vi "compare-trapezoid-profile-PID-position-ctrl.vi"() -> ()   [LabVIEW 2019]
uses:
  Secret_Control_Library_Protected/CtrlTrain_Pos_ctrl_TuningParameters.ctl
  <vilib>/Rock Robotics/WPI/ThirdParty/JAS_Junk/TrajLib/SlewRateLimiter_New.vi
  <vilib>/Rock Robotics/WPI/ThirdParty/JAS_Junk/TrajLib/SlewRateLimiter_Reset.vi
  <vilib>/Rock Robotics/WPI/ThirdParty/JAS_Junk/TrajLib/SlewRateLimiter_Calculate.vi
  <vilib>/Rock Robotics/WPI/ThirdParty/JAS_Junk/TrajLib/SlewRateLimiter_SetRate.vi
  <vilib>/Rock Robotics/WPI/ThirdParty/JAS_Junk/TrajLib/ProfiledPIDController_SetPID.vi
  <vilib>/Rock Robotics/WPI/ThirdParty/JAS_Junk/TrajLib/ProfiledPIDController_SetIntegratorRange.vi
  <vilib>/Rock Robotics/WPI/ThirdParty/JAS_Junk/TrajLib/ProfiledPIDController_SetTolerance_PosVel.vi
  <vilib>/Rock Robotics/WPI/ThirdParty/JAS_Junk/TrajLib/ProfiledPIDController_DisableContInput.vi
  <vilib>/Rock Robotics/WPI/ThirdParty/JAS_Junk/TrajLib/ProfiledPIDController_EnableContInput.vi
  <vilib>/Rock Robotics/WPI/ThirdParty/JAS_Junk/TrajLib/ProfiledPIDController_Reset_PosOnly.vi
  <vilib>/Rock Robotics/WPI/ThirdParty/JAS_Junk/TrajLib/ProfiledPIDController_NewPeriod.vi
  <vilib>/Rock Robotics/WPI/ThirdParty/JAS_Junk/TrajLib/ProfiledPIDController_Calculate_Meas_Goal.vi
  <vilib>/Rock Robotics/WPI/ThirdParty/JAS_Junk/TrajLib/ProfiledPIDController_AtGoal.vi
  <vilib>/Rock Robotics/WPI/ThirdParty/JAS_Junk/TrajLib/ProfiledPIDController_AtSetpoint.vi
  <vilib>/Rock Robotics/WPI/ThirdParty/JAS_Junk/TrajLib/ProfiledPIDController_SetConstraints.vi
  <vilib>/Rock Robotics/WPI/ThirdParty/JAS_Junk/TrajLib/Util_GetTime.vi
  <vilib>/Rock Robotics/WPI/ThirdParty/JAS_Junk/TrajLib/PIDController_SetPID.vi
  <vilib>/Rock Robotics/WPI/ThirdParty/JAS_Junk/TrajLib/PIDController_SetIntegratorRange.vi
  <vilib>/Rock Robotics/WPI/ThirdParty/JAS_Junk/TrajLib/PIDController_SetTolerancePandV.vi
  <vilib>/Rock Robotics/WPI/ThirdParty/JAS_Junk/TrajLib/PIDController_DisableContinousInput.vi
  <vilib>/Rock Robotics/WPI/ThirdParty/JAS_Junk/TrajLib/PIDController_EnableContinousInput.vi
  <vilib>/Rock Robotics/WPI/ThirdParty/JAS_Junk/TrajLib/TrapProfState_New.vi
  <vilib>/Rock Robotics/WPI/ThirdParty/JAS_Junk/TrajLib/ProfiledPIDController_Reset.vi
  <vilib>/Rock Robotics/WPI/ThirdParty/JAS_Junk/TrajLib/PIDController_NewPeriod.vi
  <vilib>/Rock Robotics/SystemInterfaces/NetworkCommunication/NetComm_UsageReport_report.vi
  <vilib>/Rock Robotics/WPI/ThirdParty/JAS_Junk/TrajLib/ProfiledPIDController_SetGoal_PosOnly.vi
  <vilib>/Rock Robotics/WPI/ThirdParty/JAS_Junk/TrajLib/ProfiledPIDController_Calculate_Meas.vi
  <vilib>/Rock Robotics/WPI/ThirdParty/JAS_Junk/TrajLib/TrapProfState_Equals.vi
  <vilib>/Rock Robotics/WPI/ThirdParty/JAS_Junk/TrajLib/PIDController_AtSetpoint.vi
  <vilib>/Rock Robotics/WPI/ThirdParty/JAS_Junk/TrajLib/VI/Util_GetTime_U32.vi
  <vilib>/Rock Robotics/WPI/ThirdParty/JAS_Junk/TrajLib/PIDController_Reset.vi
  <vilib>/Rock Robotics/WPI/ThirdParty/JAS_Junk/TrajLib/ProfiledPIDController_SetGoal.vi
  <vilib>/Rock Robotics/WPI/ThirdParty/JAS_Junk/TrajLib/PIDController_Calculate_SP_PV.vi
  <vilib>/Rock Robotics/WPI/ThirdParty/JAS_Junk/TrajLib/TrapProfile_New.vi
  <vilib>/Rock Robotics/WPI/ThirdParty/JAS_Junk/TrajLib/ProfiledPIDController_GetPeriod.vi
  <vilib>/Rock Robotics/WPI/ThirdParty/JAS_Junk/TrajLib/TrapProfile_Calculate.vi
  <vilib>/Rock Robotics/WPI/ThirdParty/JAS_Junk/TrajLib/ControllerUtil_GetModulusError.vi
  <vilib>/Rock Robotics/WPI/ThirdParty/JAS_Junk/TrajLib/PIDController_SetSetpoint.vi
  <vilib>/Rock Robotics/WPI/ThirdParty/JAS_Junk/TrajLib/PIDController_Calculate_PV.vi
  <vilib>/Rock Robotics/WPI/ThirdParty/JAS_Junk/TrajLib/TrapProfile_ShouldFlipAcceleration.vi
  <vilib>/Rock Robotics/WPI/ThirdParty/JAS_Junk/TrajLib/TrapProfile_Direct.vi
  <vilib>/Rock Robotics/WPI/ThirdParty/JAS_Junk/TrajLib/PIDController_GetPeriod.vi
  <vilib>/addons/control/pid/pid.llb/PID Lead-Lag (DBL).vi
  <vilib>/Rock Robotics/WPI/ThirdParty/JAS_Junk/TrajLib/Globals/Util_LibraryGlobals.vi
  <vilib>/Rock Robotics/WPI/ThirdParty/JAS_Junk/TrajLib/VI/Util_GetTime_U64.vi
  <vilib>/addons/control/pid/NI_PID_pid.lvlib
  Secret_Control_Library_Protected/Secret_Control_Library_Protected.lvlib
  <vilib>/Rock Robotics/WPI/ThirdParty/JAS_Junk/TrajLib/Trajectory_Library.lvlib
panel:
  in  "Tab Control":T1(tab)
  out "PC-SP, PV, CO Chart":T2(graph)
  in  "Desired Position":dbl(slide) min=0.0 max=90.0 scale=0.0..90.0
  in  "Auto - Set Position To 0 / Manual - Lower":bool
  in  "Auto - Set Position to 90 / Manual - Raise":bool
  in  "Set Position to Desired\n(Select to activate position)":bool
  out "Selected Setpoint \n(In Manual \ntracks Position)":dbl
  out "Trap-Current \nPosition 2":dbl format="%.2f"
  out "Trap-Motor \nDemand2":dbl format="%#.2f"
  out "Trap-Position Error":dbl format="%#3.2f"
  out "Trap-SP, PV, CO Chart":T2(graph)
  out "Trap-Current Position":dbl(knob) scale=-10.0..100.0
  in  "Auto / Manual":bool=TRUE
  in  "MinLimitSwitch":bool
  in  "MaxLimitSwitch":bool
  out "Trap-In Position":bool
  out "PC-Current \nPosition 2":dbl format="%.2f"
  out "PC-Motor \nDemand 2":dbl format="%#.2f"
  out "PC-Current Position 3":dbl(knob) scale=-10.0..100.0
  out "Selected Setpoint \n(In Manual \ntracks Position) 2":dbl
  out "PC-In Position":bool
  out "PC-Position Error":dbl format="%#3.2f"
  in  "MaxLimitSwitch 2":bool
  in  "MinLimitSwitch 2":bool
  out "AtGoal":bool
  in  "Trap-Max Accel":dbl=18.0 format="%#_13g"
  in  "PC-TuningParameters":T3={"MaxOutput"=1.0, "MinOutput"=0.25, "PositionErrThreshold"=6.0, "PositionErrDeadband"=0.5, "ReverseOutput"=FALSE, "PositionMax"=89.0, "PositionMin"=1.0, "WithinDBCount"=5} {"WithinDBCount" min=1}
  in  "trap-PositionTolerance":dbl=0.5 format="%#_13g"
  in  "Trap-VelocityTolerance":dbl=1.0 format="%#_13g"
  in  "Trap-ConsecutiveAtGoalCount":i32=5
  in  "Trap-Max Speed":dbl=8.5 format="%#_13g"
  in  "PC-MaxAccelRate":dbl=1.4 format="%#_13g"
  in  "Output Deadband":dbl=0.08 format="%#_13g"
  in  "At Reference Count":i32=10
  in  "Max Allowd Position":dbl=89.0 format="%#_13g"
  in  "Min Allowd Position":dbl=1.0 format="%#_13g"
  in  "ErrorThreshold":dbl=6.5 format="%#_13g"
  in  "MaxOutput":dbl=1.0 format="%#_13g"
  in  "Output Threshold":dbl=1.0 format="%#_13g"
  in  "ErrorDeadband":dbl=0.5 format="%#_13g"
  in  "Kp":dbl=1.5 format="%#_13g"
  out "Both-Current-Setpoint":dbl
  out "Trap-Current-Position":dbl
  out "Both-Manual-Lower":bool
  out "Both-Manual-Raise":bool
  out "Trap-Motor-Demand":dbl
  out "PC-Current-Position":dbl
  out "PC-Motor-Demand":dbl
  # "Compare trapezoid with position control"
  # "Toggle these switches to simulate a limit switch input."
  # "Trapezoid Profile"
  # "Position Control"
  # "Max Vel = 8.5"
  # "Max Output = 1.0"
  # "1.25"
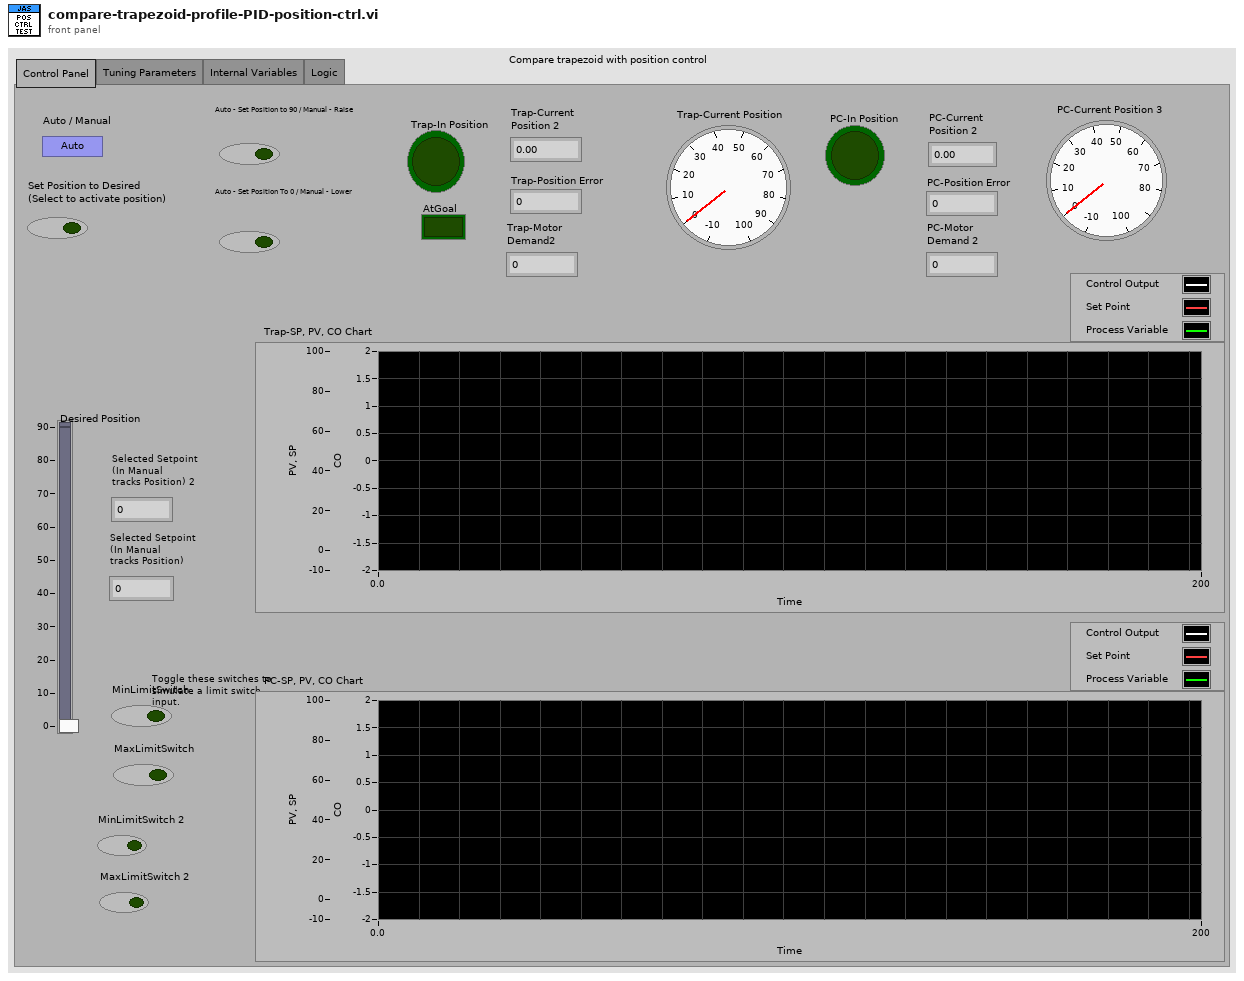
[diagram p1: front panel]
types:
  T1 = enum32{"Control Panel", "Tuning Parameters", "Internal Variables", "Logic"}
  T2 = cluster{"MotorDemand":dbl, "CurrentSetpoint":dbl, "CurrentPosition":dbl}
  T3 = typedef "Secret_Control_Library_Protected.lvlib/CtrlTrain_Pos_ctrl_TuningParameters.ctl" = cluster{"MaxOutput":dbl, "MinOutput":dbl, "PositionErrThreshold":dbl, "PositionErrDeadband":dbl, "ReverseOutput":bool, "PositionMax":dbl, "PositionMin":dbl, "WithinDBCount":i32}
  T4 = cluster{"gain":dbl, "lag time":dbl, "lead time":dbl}
  T5 = cluster{"PC-Motor-Demand":dbl, "Both-Current-Setpoint":dbl, "PC-Current-Position":dbl}
  T6 = typedef "Trajectory_Library.lvlib/PID_TUNING.ctl" = cluster{"Kp":dbl, "Ki":dbl, "Kd":dbl, "MaximumIntegral":dbl, "MinimumIntegral":dbl}
  T7 = typedef "Trajectory_Library.lvlib/PID_INPUT_LIMITS.ctl" = cluster{"MaxInput":dbl, "MinInput":dbl, "Continuous":bool}
  T8 = typedef "Trajectory_Library.lvlib/TRAPEZOID_PROFILE_CONSTRAINT.ctl" = cluster{"MaxVelocity":dbl, "MaxAcceleration":dbl}
  T9 = typedef "Trajectory_Library.lvlib/PID_ERROR_TOLERANCE.ctl" = cluster{"PositionTolerance":dbl, "VelocityTolerance":dbl}
  T10 = typedef "Trajectory_Library.lvlib/PROFILED_PID_CONTROLLER.ctl" = cluster{"Controller":T11, "Goal":T12, "Setpoint":T12, "Constraint":T8}
  T11 = typedef "Trajectory_Library.lvlib/PID_CONTROLLER.ctl" = cluster{"Kp":dbl, "Ki":dbl, "Kd":dbl, "Period":dbl, "Max_Integral":dbl, "Min_Integral":dbl, "Max_Input":dbl, "Min_Input":dbl, "Continuous":bool, "PositionError":dbl, "VelocityError":dbl, "PrevError":dbl, "TotalError":dbl, "PositionTolerance":dbl, "VelocityTolerance":dbl, "SetPoint":dbl, "Kf":dbl, "Prev_Deriv":dbl, "Prev_Deriv 2":dbl, "DerivativeFilter":bool, "Min_Output":dbl, "Max_Output":dbl, "Prev_F_P":dbl, "Prev_F_P_2":dbl, "AntiWindupActive":bool, "Measurement":dbl}
  T12 = typedef "Trajectory_Library.lvlib/TRAPEZOID_PROFILE_STATE.ctl" = cluster{"Position":dbl, "Velocity":dbl}
  T13 = cluster{"Trap-Motor-Demand":dbl, "Both-Current-Setpoint":dbl, "Trap-Current-Position":dbl}
  T14 = typedef "Trajectory_Library.lvlib/PosCtrl_Tuning_Type.ctl" = cluster{"Slope":dbl, "Offset":dbl, "Error Deadband":dbl, "At Reference Count":i32, "Negate Output":bool, "Max Allowd Position":dbl, "Min Allowd Position":dbl}
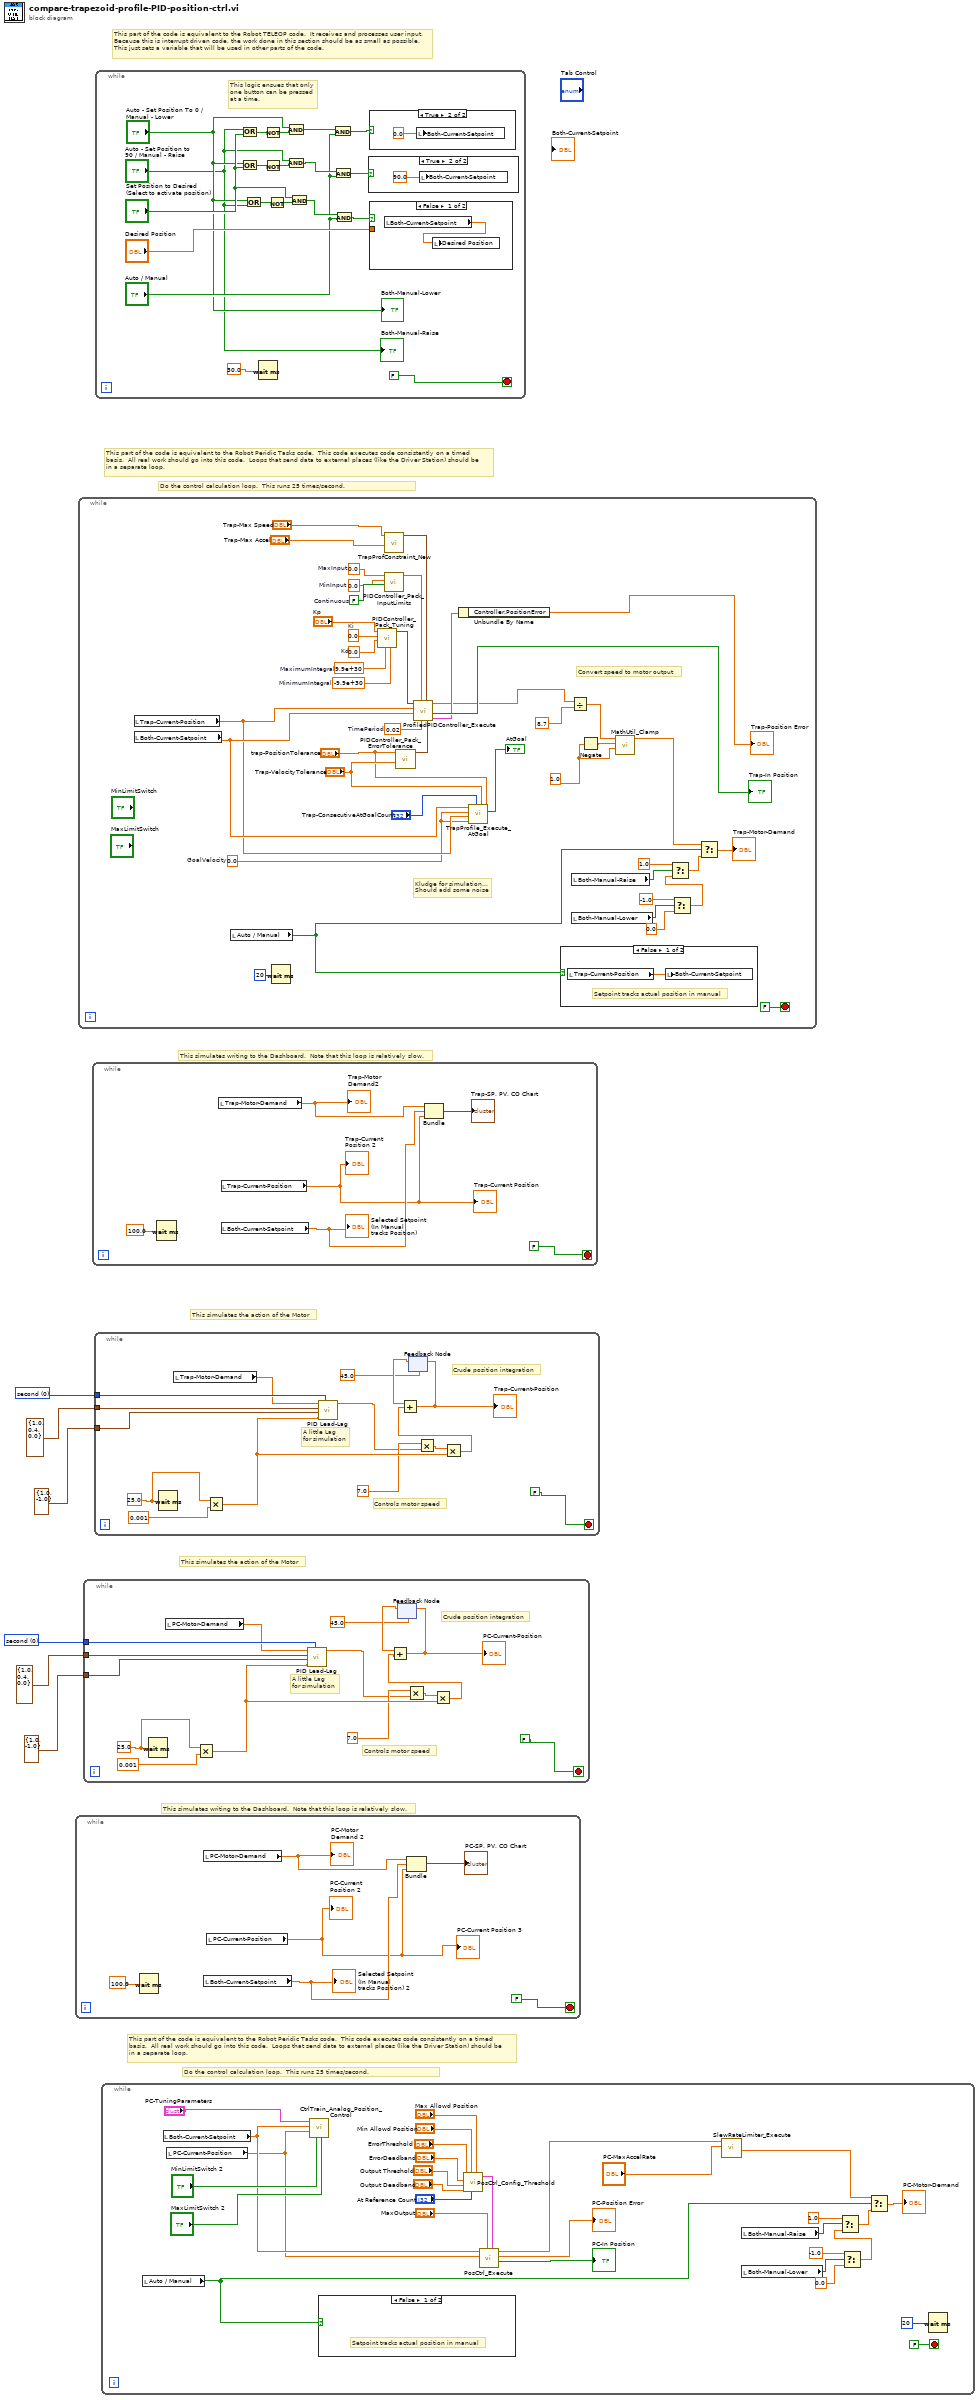
[diagram p0: block diagram]
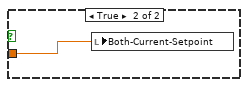
[diagram p4: hidden frame]
diagram:
  w1 = u16 0 items=["second", "minute"] ("time unit")
  w6 = u16 0 items=["second", "minute"] ("time unit")
  # "Do the control calculation loop.  This runs 25 times/second."
  # "This part of the code is equivalent to the Robot Peridic Tasks code.  This code executes code consistently on a timed\nbasis.  All real work should go into this code.  Loops that send data to external places (like the Driver Station) should be \nin a separate loop."
  # "This simulates writing to the Dashboard.  Note that this loop is relatively slow."
  # "This simulates the action of the Motor"
  # "This simulates the action of the Motor"
  # "This simulates writing to the Dashboard.  Note that this loop is relatively slow."
  # "Do the control calculation loop.  This runs 25 times/second."
  # "This part of the code is equivalent to the Robot Peridic Tasks code.  This code executes code consistently on a timed\nbasis.  All real work should go into this code.  Loops that send data to external places (like the Driver Station) should be \nin a separate loop."
  # "This part of the code is equivalent to the Robot TELEOP code.  It receives and processes user input.\nBecause this is interrupt driven code, the work done in this section should be as small as possible.\nThis just sets a variable that will be used in other parts of the code."
  n1 = while {
    stop <- FALSE stop-if-true
    n2 = Wait (ms)(milliseconds to wait=100.0) -> ()  [unwired: 1 out]
    n3 = local read "PC-Motor-Demand"() -> (w8:dbl)
    "PC-Motor \nDemand 2" <- w8
    n4 = local read "Both-Current-Setpoint"() -> (w10:dbl)
    "Selected Setpoint \n(In Manual \ntracks Position) 2" <- w10
    n5 = local read "PC-Current-Position"() -> (w9:dbl)
    "PC-Current \nPosition 2" <- w9
    "PC-Current Position 3" <- w9
    n6 = Bundle("PC-Motor-Demand"=w8, "Both-Current-Setpoint"=w10, "PC-Current-Position"=w9) -> (→"PC-SP, PV, CO Chart":T5)  [unwired: 1 in]
  }
  n7 = while {
    stop <- FALSE stop-if-true
    w23 = 1.0
    w37 = 0.0  # MaxInput
    w38 = 0.0  # MinInput
    w39 = FALSE  # Continuous
    w33 = 0.0  # Ki
    w34 = 0.0  # Kd
    w35 = 9.9e+30  # MaximumIntegral
    w36 = -9.9e+30  # MinimumIntegral
    w13 = 0.0  # GoalVelocity
    w31 = 0.02  # TimePeriod
    # "Convert speed to motor output"
    # "Kludge for simulation...\nShould add some noise"
    n8 = local read "Trap-Current-Position"() -> (w15:dbl)
    n9 = local read "Both-Current-Setpoint"() -> (w16:dbl)
    n10 = local read "Auto / Manual"() -> (w49:bool)
    n11 = Wait (ms)(milliseconds to wait=u32 20) -> ()  [unwired: 1 out]
    n12 = call <vilib>:"PIDController_Pack_Tuning.vi"("MinimumIntegral"=w36, "MaximumIntegral"=w35, "Kd"=w34, "Ki"=w33, "Kp"="Kp") -> ("PID Tuning"=w41:T6)  [unwired: 6 in]
    n13 = call <vilib>:"PIDController_Pack_InputLimits.vi"("Continuous"=w39, "MinInput"=w38, "MaxInput"=w37) -> ("PID Input Limits"=w42:T7)  [unwired: 8 in]
    n14 = call <vilib>:"TrapProfConstraint_New.vi"("Max Accel"="Trap-Max Accel", "Max Speed (M/S)"="Trap-Max Speed") -> ("TRAPEZOID_PROFILE_CONSTRAINT"=w40:T8)  [unwired: 9 in]
    n15 = call <vilib>:"PIDController_Pack_ErrorTolerance.vi"("VelocityTolerance"="Trap-VelocityTolerance", "PositionTolerance"="trap-PositionTolerance") -> ("PID Error Tolerance"=w30:T9)  [unwired: 9 in]
    n16 = call <vilib>:"ProfiledPIDController_Execute.vi"("PID Error Tolerance"=w30, "Constraints"=w40, "Period"=w31, "PID Input Limits"=w42, "SP-SetPoint Goal"=w16, "PV-Measurement"=w15, "PID Tuning"=w41) -> ("out PID_CONTROLLER"=w27:T10, "AtSetpoint"=→"Trap-In Position":bool, "CO-ControlOutput"=w22:dbl)  [unwired: 1 in, 1 out]
    n17 = Unbundle By Name(w27) -> ("Controller.PositionError"=→"Trap-Position Error":dbl)
    n18 = call <vilib>:"TrapProfile_Execute_AtGoal.vi"("PositionTolerance"="trap-PositionTolerance", "VelocityTolerance"="Trap-VelocityTolerance", "ConsecutiveAtGoalCount"="Trap-ConsecutiveAtGoalCount", "CurrentVelocity"=w13, "CurrentPosition"=w15, "GoalVelocity"=w13, "GoalPosition"=w16) -> ("AtGoal"=→"AtGoal":bool)  [unwired: 4 in]
    n19 = case shown="False" w49 {
      frame False {
        # "Setpoint tracks actual position in manual"
        n20 = local read "Trap-Current-Position"() -> (w55:dbl)
        n21 = local write "Both-Current-Setpoint"(w55) -> ()
      }
      frame True {
      }
    }
    n22 = Divide(x=w22, y=8.7) -> (x/y=w21:dbl)
    n23 = local read "Both-Manual-Raise"() -> (w48:bool)
    n24 = local read "Both-Manual-Lower"() -> (w47:bool)
    n25 = Negate(x=w23) -> (-x=w25:dbl)
    n26 = call <vilib>:"MathUtil_Clamp.vi"("High Limit"=w23, "Low Limit"=w25, "Value"=w21) -> ("Result"=w20:dbl)  [unwired: 8 in]
    n27 = Select(t=-1.0, s=w47, f=0.0) -> (s? t:f=w51:dbl)
    n28 = Select(t=1.0, s=w48, f=w51) -> (s? t:f=w50:dbl)
    n29 = Select(t=w20, s=w49, f=w50) -> (s? t:f=→"Trap-Motor-Demand":dbl)
  }
  n30 = while {
    tunnel: w1 -> [w70]
    tunnel: T4 {"gain"=1.0, "lag time"=0.4, "lead time"=0.0} ("tuning parameters") -> [w69]
    tunnel: cluster{"output high":dbl, "output low":dbl} {"output high"=1.0, "output low"=-1.0} ("output range") -> [w67]
    stop <- FALSE stop-if-true
    w59 = 25.0
    # "Controls motor speed"
    # "Crude position integration"
    # "A little Lag\nfor simulation"
    n31 = Wait (ms)(milliseconds to wait=w59) -> ()  [unwired: 1 out]
    n32 = local read "PC-Motor-Demand"() -> (w56:dbl)
    n33 = Multiply(x=w59, y=0.001) -> (x*y=w66:dbl)
    n34 = call-poly <vilib>:"PID Lead-Lag.vi"("time unit"=w70, "dt (s)"=w66, "output range"=w67, "tuning parameters"=w69, "input"=w56) -> ("output"=w58:dbl)  [unwired: 3 in, 1 out]
    n35 = feedback #1(45.0) -> (w64:dbl)
    n36 = Multiply(x=7.0, y=w58) -> (x*y=w65:dbl)
    n37 = Multiply(x=w65, y=w66) -> (x*y=w62:dbl)
    n38 = Add(x=w64, y=w62) -> (x+y=w57:dbl)
    "PC-Current-Position" <- w57
    n39 = feedback-in #1(w57) -> ()
  }
  n40 = while {
    stop <- FALSE stop-if-true
    n41 = Wait (ms)(milliseconds to wait=100.0) -> ()  [unwired: 1 out]
    n42 = local read "Trap-Motor-Demand"() -> (w71:dbl)
    "Trap-Motor \nDemand2" <- w71
    n43 = local read "Trap-Current-Position"() -> (w72:dbl)
    "Trap-Current \nPosition 2" <- w72
    "Trap-Current Position" <- w72
    n44 = local read "Both-Current-Setpoint"() -> (w73:dbl)
    "Selected Setpoint \n(In Manual \ntracks Position)" <- w73
    n45 = Bundle("Trap-Motor-Demand"=w71, "Both-Current-Setpoint"=w73, "Trap-Current-Position"=w72) -> (→"Trap-SP, PV, CO Chart":T13)  [unwired: 1 in]
  }
  n46 = while {
    tunnel: w6 -> [w91]
    tunnel: T4 {"gain"=1.0, "lag time"=0.4, "lead time"=0.0} ("tuning parameters") -> [w90]
    tunnel: cluster{"output high":dbl, "output low":dbl} {"output high"=1.0, "output low"=-1.0} ("output range") -> [w88]
    stop <- FALSE stop-if-true
    w80 = 25.0
    # "Controls motor speed"
    # "Crude position integration"
    # "A little Lag\nfor simulation"
    n47 = Wait (ms)(milliseconds to wait=w80) -> ()  [unwired: 1 out]
    n48 = local read "Trap-Motor-Demand"() -> (w77:dbl)
    n49 = Multiply(x=w80, y=0.001) -> (x*y=w87:dbl)
    n50 = call-poly <vilib>:"PID Lead-Lag.vi"("time unit"=w91, "dt (s)"=w87, "output range"=w88, "tuning parameters"=w90, "input"=w77) -> ("output"=w79:dbl)  [unwired: 3 in, 1 out]
    n51 = feedback #2(45.0) -> (w85:dbl)
    n52 = Multiply(x=7.0, y=w79) -> (x*y=w86:dbl)
    n53 = Multiply(x=w86, y=w87) -> (x*y=w83:dbl)
    n54 = Add(x=w85, y=w83) -> (x+y=w78:dbl)
    "Trap-Current-Position" <- w78
    n55 = feedback-in #2(w78) -> ()
  }
  n56 = while {
    stop <- FALSE stop-if-true
    # "This logic ensues that only\none button can be pressed\nat a time."
    n57 = Or(x="Auto - Set Position to 90 / Manual - Raise", y="Set Position to Desired\n(Select to activate position)") -> (x .or. y?=w110:bool)
    n58 = Or(x="Auto - Set Position To 0 / Manual - Lower", y="Set Position to Desired\n(Select to activate position)") -> (x .or. y?=w108:bool)
    n59 = Or(x="Auto - Set Position To 0 / Manual - Lower", y="Auto - Set Position to 90 / Manual - Raise") -> (x .or. y?=w106:bool)
    n60 = Wait (ms)(milliseconds to wait=30.0) -> ()  [unwired: 1 out]
    n61 = Not(x=w110) -> (.not. x?=w109:bool)
    n62 = Not(x=w108) -> (.not. x?=w107:bool)
    n63 = Not(x=w106) -> (.not. x?=w105:bool)
    n64 = And(x="Auto - Set Position To 0 / Manual - Lower", y=w109) -> (x .and. y?=w100:bool)
    n65 = And(x="Auto - Set Position to 90 / Manual - Raise", y=w107) -> (x .and. y?=w96:bool)
    n66 = And(x="Set Position to Desired\n(Select to activate position)", y=w105) -> (x .and. y?=w95:bool)
    n67 = And(x=w100, y="Auto / Manual") -> (x .and. y?=w99:bool)
    n68 = And(x=w96, y="Auto / Manual") -> (x .and. y?=w98:bool)
    n69 = And(x=w95, y="Auto / Manual") -> (x .and. y?=w97:bool)
    n70 = case shown="True" w98 {
      frame False {
      }
      frame True {
        n71 = local write "Both-Current-Setpoint"(90.0) -> ()
      }
    }
    n72 = case shown="True" w99 {
      frame False {
      }
      frame True {
        n73 = local write "Both-Current-Setpoint"(0.0) -> ()
      }
    }
    n74 = case shown="False" w97 {
      tunnel: "Desired Position" -> [_ w112]
      frame False {
        n75 = local read "Both-Current-Setpoint"() -> (w111:dbl)
        n76 = local write "Desired Position"(w111) -> ()
      }
      frame True {
        n77 = local write "Both-Current-Setpoint"(w112) -> ()
      }
    }
    "Both-Manual-Raise" <- "Auto - Set Position to 90 / Manual - Raise"
    "Both-Manual-Lower" <- "Auto - Set Position To 0 / Manual - Lower"
  }
  n78 = while {
    stop <- FALSE stop-if-true
    n79 = local read "Auto / Manual"() -> (w115:bool)
    n80 = local read "Both-Current-Setpoint"() -> (w124:dbl)
    n81 = local read "PC-Current-Position"() -> (w123:dbl)
    n82 = call "CtrlTrain_Analog_Position_Control.vi"("PositionMax"="MaxLimitSwitch 2", "PositionMin"="MinLimitSwitch 2", "CurrentPosition"=w123, "TargetPosition"=w124, "Pos_Ctrl_TuningParameters"="PC-TuningParameters") -> ()  [unwired: 4 in, 3 out]
    n83 = case shown="False" w115 {
      frame False {
        # "Setpoint tracks actual position in manual"
      }
      frame True {
      }
    }
    n84 = call <vilib>:"PosCtrl_Config_Threshold.vi"("Max Allowd Position"="Max Allowd Position", "At Reference Count"="At Reference Count", "Min Allowd Position"="Min Allowd Position", "Output Deadband"="Output Deadband", "Output Threshold"="Output Threshold", "ErrorDeadband"="ErrorDeadband", "ErrorThreshold"="ErrorThreshold") -> ("PosCtrl_Config_Params"=w129:T14)  [unwired: 4 in]
    n85 = call <vilib>:"PosCtrl_Execute.vi"("PosCtrl_Config_Params"=w129, "MaxOutput"="MaxOutput", "CurrentPosition"=w123, "TargetPosition"=w124) -> ("OnTarget"=→"PC-In Position":bool, "PositionError"=→"PC-Position Error":dbl, "Output"=w120:dbl)  [unwired: 5 in]
    n86 = call <vilib>:"SlewRateLimiter_Execute.vi"("PositiveRate"="PC-MaxAccelRate", "Input"=w120) -> ("Output"=w130:dbl)  [unwired: 8 in, 1 out]
    n87 = local read "Both-Manual-Raise"() -> (w139:bool)
    n88 = local read "Both-Manual-Lower"() -> (w138:bool)
    n89 = Select(t=-1.0, s=w138, f=0.0) -> (s? t:f=w141:dbl)
    n90 = Select(t=1.0, s=w139, f=w141) -> (s? t:f=w140:dbl)
    n91 = Select(t=w130, s=w115, f=w140) -> (s? t:f=→"PC-Motor-Demand":dbl)
    n92 = Wait (ms)(milliseconds to wait=u32 20) -> ()  [unwired: 1 out]
  }
